vi "To Serial Form.vi"(6 "Serial Version":T1, 10 "Serializer in":refnum<class "Serializer.lvclass">, 11 "Single in":refnum<class "Single.lvclass">) -> (0 "error out":errorcluster, 2 "Serializer out":refnum<class "Serializer.lvclass">, 3 "Single out":refnum<class "Single.lvclass">)   [LabVIEW 2014, in "Base Data Class.lvlib" / "Single.lvclass"]
uses:
  Single.lvclass
  <vilib>/NI/AQ Character Lineator/Serializer/Serializer.lvclass
  <vilib>/NI/AQ Character Lineator/Serialization Common/Serial Version.ctl
  Single.lvclass/Single.ctl
  <vilib>/NI/AQ Character Lineator/Serializable/Insert Single.vi
  <vilib>/NI/AQ Character Lineator/Serializer/Insert Single.vi
  <vilib>/NI/AQ Character Lineator/Serializer/Read Include Default Values.vi
  Data.lvclass
  <vilib>/NI/AQ Character Lineator/Serializable/Serializable.lvclass
  <vilib>/NI/AQ Character Lineator/Serialization Common/Serialization Common.lvlib
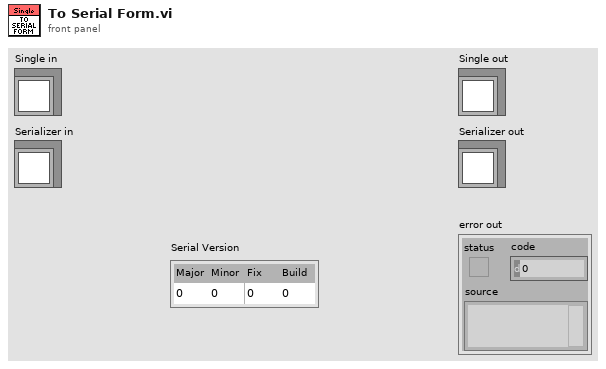
[diagram p1: front panel]
types:
  T1 = typedef "Serialization Common.lvlib/Serial Version.ctl" = cluster{"Major":u16, "Minor":u16, "Fix":u16, "Build":u16}
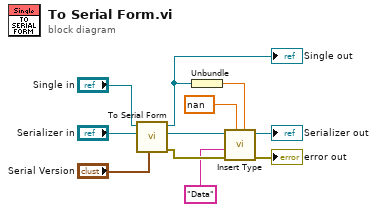
[diagram p0: block diagram]
diagram:
  n1 = call-parent "To Serial Form.vi"("Serial Version"="Serial Version", "Serializer in"="Serializer in", "Data in"="Single in") -> ("error out"=w4:errorcluster, "Serializer out"=w8:refnum<class "Serializer.lvclass">, "Data out"=w7:refnum<class "Single.lvclass">)  [unwired: 6 in]
  "Single out" <- w7
  n2 = Unbundle(w7) -> (w6:sgl)
  n3 = call-poly <vilib>:"Insert Type.vi"("Double"=w6, "Default Value"=sgl nan, "error in (no error)"=w4, "Name"="Data", "Serializer in"=w8) -> ("error out"=→"error out":errorcluster, "Serializer out"=→"Serializer out":refnum<class "Serializer.lvclass">)  [unwired: 5 in]
